vi "SUB_USBDAQ_channel_string.vi"(1 "channel":string[](array[string])) -> (2 "Device Name":string, 3 "IsDevFind":bool, 4 "resulting string":string)   [LabVIEW 2011]
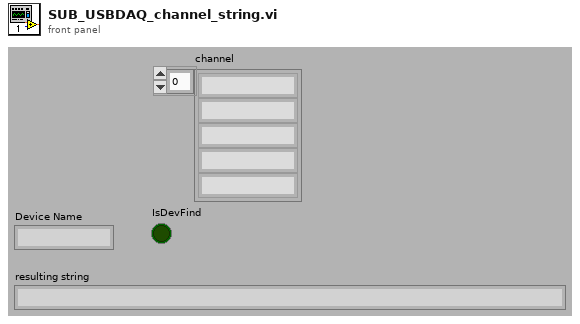
[diagram p1: front panel]
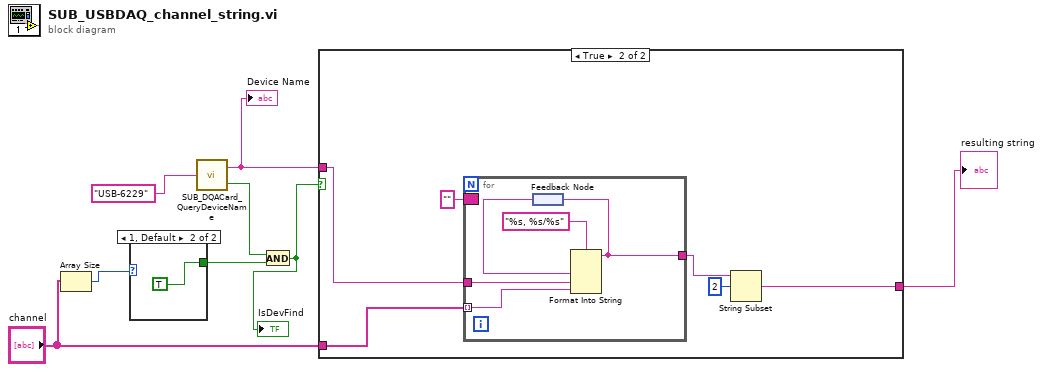
[diagram p0: block diagram]
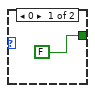
[diagram p2: hidden frame]
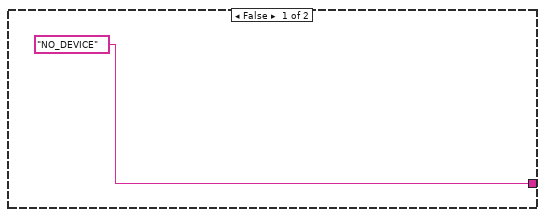
[diagram p3: hidden frame]
diagram:
  n1 = Array Size(array="channel") -> (size(s)=w2:i32)
  n2 = case shown="1, Default" w2 {
    tunnel: [FALSE TRUE] -> w1
    frame 0 {
    }
    frame 1, Default {
    }
  }
  n3 = call "SUB_DQACard_QueryDeviceName.vi"("Search device type"="USB-6229") -> ("Device Name"=w7:string, "Find?"=w4:bool)
  "Device Name" <- w7
  n4 = And(x=w4, y=w1) -> (x .and. y?=w3:bool)
  "IsDevFind" <- w3
  n5 = case shown="True" w3 {
    tunnel: w7 -> [_ w16]
    tunnel: "channel" -> [_ w17]
    tunnel: ["NO_DEVICE" w13] -> w6
    frame False {
    }
    frame True {
      n6 = for {
        tunnel: w17 -> [w21] mode=indexing
        tunnel: w16 -> [w20]
        tunnel: [w18] -> w15
        border: "" -> [_]
        n7 = feedback #1() -> (w19:string)
        n8 = Format Into String(format string="%s, %s/%s", w19, w20, w21) -> (resulting string=w18:string)  [unwired: 2 in, 1 out]
        n9 = feedback-in #1(w18) -> ()
      }
      n10 = String Subset(string=w15, offset (0)=2) -> (substring=w13:string)  [unwired: 1 in]
    }
  }
  "resulting string" <- w6
